vi "Log Message core.vi"(7 "Time Stamp":timestamp, 8 "error in (no error)":errorcluster, 9 "Message":refnum<class "Message.lvclass">, 10 "Receiving Actor":refnum<class "Message Enqueuer.lvclass">, 11 "Monitor Window in":refnum<class "Classic Monitor.lvclass">) -> (0 "error out":errorcluster, 3 "Monitor Window out":refnum<class "Classic Monitor.lvclass">)   [LabVIEW 2017, in "MGI-Monitored Actor.lvlib" / "Classic Monitor.lvclass"]
uses:
  Classic Monitor.lvclass
  <vilib>/ActorFramework/Message/Message.lvclass
  <vilib>/ActorFramework/Message Enqueuer/Message Enqueuer.lvclass
  Classic Monitor.lvclass/Classic Monitor.ctl
  Logger/Logger Messages/New Message Msg/New Message Msg.lvclass
  monitored-actor-core/Source/Monitored Actor/Monitored Actor Messages/Disable Message Logging Msg/Disable Message Logging Msg.lvclass
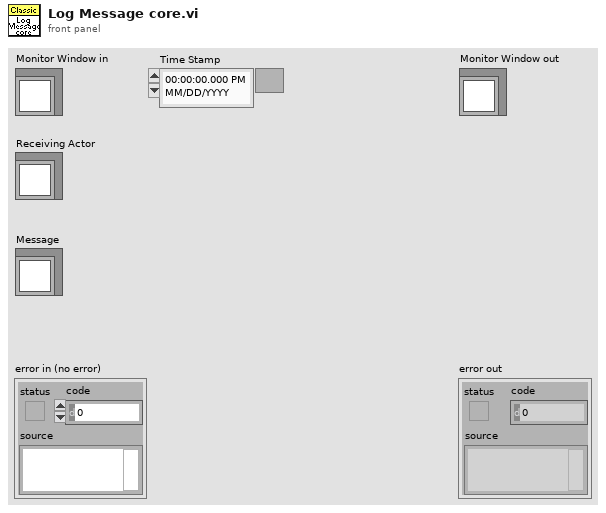
[diagram p1: front panel]
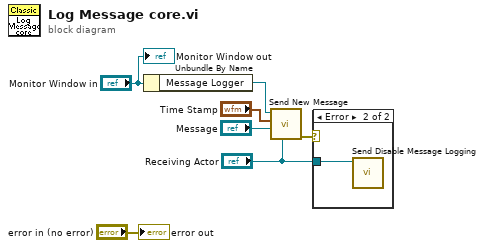
[diagram p0: block diagram]
diagram:
  n1 = Unbundle By Name("Monitor Window in") -> ("Message Logger"=w5:refnum<class "Message Enqueuer.lvclass">)
  n2 = call "Send New Message.vi"("Receiving Actor"="Receiving Actor", "Message"="Message", "Time Stamp"="Time Stamp", "Message Enqueuer in"=w5) -> ("error out"=w2:errorcluster)  [unwired: 6 in, 1 out]
  n3 = case shown="Error" w2 {
    tunnel: "Receiving Actor" -> [_ w8]
    frame No Error {
    }
    frame Error {
      n4 = call "Send Disable Message Logging.vi"("Message Enqueuer in"=w8) -> ()  [unwired: 9 in, 2 out]
    }
  }
  "error out" <- "error in (no error)"
  "Monitor Window out" <- "Monitor Window in"
